vi "10TW_PowerMode.vi"() -> ()   [LabVIEW 2013]
uses:
  shared programs/GUI_Template/GUI_master/tcp new data cluster.ctl
panel:
  in  "Position.Channel 15::1":bool caption="X-Hair #1"
  in  "Position.Channel 14::1":bool caption="X-Hair #5"
  in  "Position.Channel 13::1":bool caption="X-Hair #4"
  in  "Position.Channel 12::1":bool caption="X-Hair #3"
  in  "Position.Channel 11::1":bool=TRUE caption="X-Hair #2"
  in  "Position.Channel 10::1":bool caption="Int X-Hair"
  in  "Position.Channel 9::1":bool caption="X-Hair #0"
  in  "Position.Channel 6::1":bool caption="Mirror #10"
  in  "Position.Channel 5::1":bool caption="SSA Pickoff"
  in  "stop":bool
  in  "GUIdevice 1":string="Flipper_Controller"
  in  "insert tag":bool=TRUE
  # "10TW Alignment Targets"
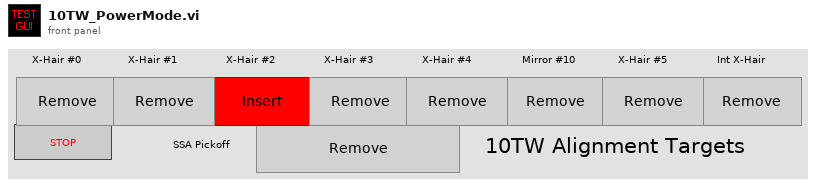
[diagram p1: front panel]
types:
  T1 = typedef "tcp new data cluster.ctl" = cluster{"EventEnum":enum16{"new data", "connection status update"}, "Device name":string}
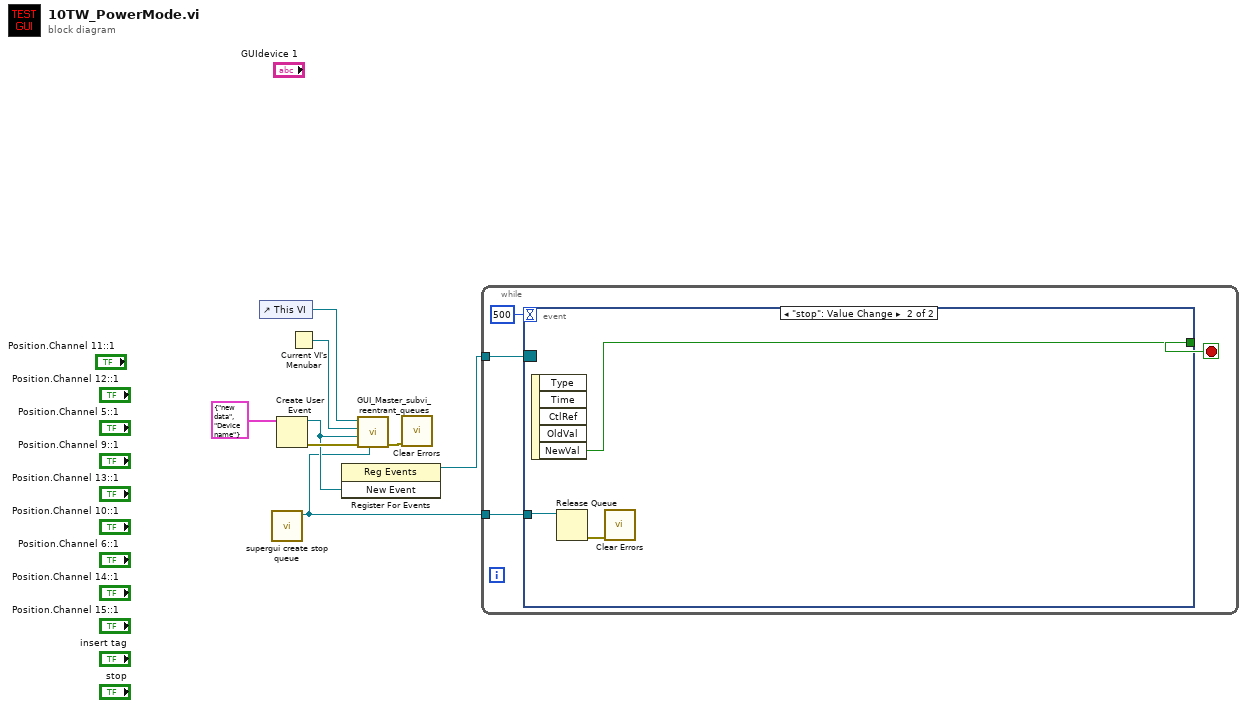
[diagram p0: block diagram]
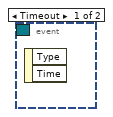
[diagram p2: hidden frame]
diagram:
  n1 = control-ref of="This VI"() -> (w8:refnum<vi>)
  n2 = call "supergui create stop queue.vi"() -> ("STOP Queue out"=w1:refnum<queue>)  [unwired: 11 in]
  n3 = Create User Event(user event datatype=T1 {"EventEnum"=enum."new data", "Device name"="Device name"} ("New Event")) -> (user event=w3:refnum<user-event>, error out=w5:errorcluster)  [unwired: 1 in]
  n4 = Current VI's Menubar() -> (w7:refnum<k9>)
  n5 = register-events(w3) -> (reference out=w2:refnum<event-registration>)  [unwired: 2 in, 1 out]
  n6 = call "GUI_Master_subvi_reentrant_queues.vi"("STOP Queue in"=w1, "error in (no error)"=w5, "tcp data event"=w3, "Caller menu reference"=w7, "Caller VI ref"=w8) -> ("error out"=w4:errorcluster)  [unwired: 6 in]
  n7 = call <vilib>:"Clear Errors.vi"("error in (no error)"=w4) -> ()  [unwired: 6 in, 1 out]
  n8 = while {
    tunnel: w2 -> [w12]
    tunnel: w1 -> [w9]
    stop <- w11 stop-if-true
    n9 = event shown="[1] \"stop\": Value Change" {
      selector: w12 -> [_ _]
      dyn-events: _ -> [_ _]
      timeout: 500 -> [_ _]
      tunnel: [_ w15] -> w11
      tunnel: w9 -> [_ w14]
      event Timeout {
        n10 = event-data() -> ()  [unwired: 1 in, 2 out]
      }
      event "stop": Value Change {
        n11 = event-data() -> ("NewVal"=w15:bool)  [unwired: 1 in, 4 out]
        n12 = Release Queue(queue=w14) -> (error out=w13:errorcluster)  [unwired: 2 in, 2 out]
        n13 = call <vilib>:"Clear Errors.vi"("error in (no error)"=w13) -> ()  [unwired: 6 in, 1 out]
      }
    }
  }
